vi "store_time_start.vi"() -> ()   [LabVIEW 2021]
panel:
  in  "error in (no error)":errorcluster
  in  "VISA resource name":refnum<visa-resource-name>
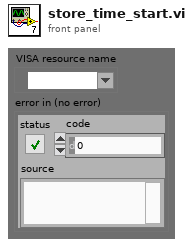
[diagram p1: front panel]
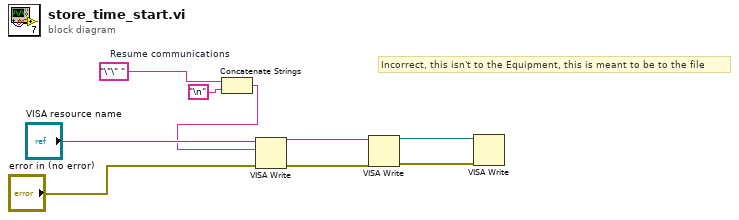
[diagram p0: block diagram]
diagram:
  w7 = "\"\" "  # Resume communications
  # "Incorrect, this isn't to the Equipment, this is meant to be to the file"
  n1 = Concatenate Strings(w7, "\n") -> (w5:string)
  n2 = VISA Write(VISA resource name="VISA resource name", write buffer=w5, error in (no error)="error in (no error)") -> (VISA resource name out=w1:refnum<visa-resource-name>, error out=w4:errorcluster)  [unwired: 1 out]
  n3 = VISA Write(VISA resource name=w1, error in (no error)=w4) -> (VISA resource name out=w2:refnum<visa-resource-name>, error out=w3:errorcluster)  [unwired: 1 in, 1 out]
  n4 = VISA Write(VISA resource name=w2, error in (no error)=w3) -> ()  [unwired: 1 in, 3 out]
